vi "NTV_Drive_Tele Balance Speed.vi"(7 "Read(f) Write(t)":bool, 11 "Balance Speed":dbl=10.0) -> (3 "Balance Speed":dbl)   [LabVIEW 2020]
uses:
  <vilib>/Rock Robotics/Network Tables/NT Read Number.vi
  <vilib>/Rock Robotics/Network Tables/NT Write Number.vi
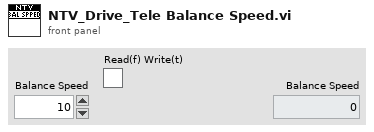
[diagram p1: front panel]
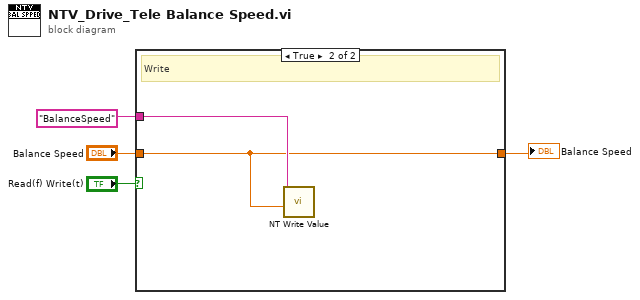
[diagram p0: block diagram]
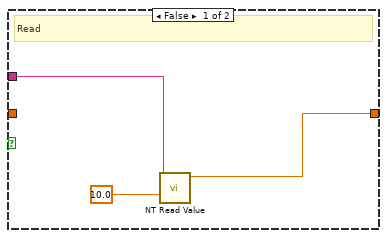
[diagram p2: hidden frame]
diagram:
  n1 = case shown="True" "Read(f) Write(t)" {
    tunnel: "Balance Speed" -> [_ w8]
    tunnel: "BalanceSpeed" ("Name") -> [w7 w9]
    tunnel: [w6 w8] -> w1
    frame False {
      # "Read"
      n2 = call-poly <vilib>:"NT Read Value.vi"("default value"=10.0, "name"=w7) -> ("value"=w6:dbl)  [unwired: 7 in, 2 out]
    }
    frame True {
      # "Write"
      n3 = call-poly <vilib>:"NT Write Value.vi"("value"=w8, "name"=w9) -> ()  [unwired: 9 in, 1 out]
    }
  }
  "Balance Speed" <- w1
